vi "Teleop.vi"(10 "Match Info":T1={"Autonomous Elapsed Seconds"=0.0, "TeleOp Elapsed Seconds"=0.0, "Disabled Elapsed Seconds"=0.0, "Visited Autonomous"=FALSE, "Visited TeleOp"=FALSE, "Visited Disabled"=FALSE, "Autonomous Settings"={"Autonomous Style"=enum."Independent", "VI Refnum"=refnum}}, 11 "Call Context":T2) -> ()   [LabVIEW 2011]
doc: "This VI is called for each TeleOp packet received from the DS where the robot is not disabled. It is often used to read from the joysticks and update I/O or to update setpoints for timed control loops. It should complete and return within 20 milliseconds or it may miss DS packets."
uses:
  <vilib>/Rock Robotics/WPI/DriverStation/WPI_DriverStationDerivedRobotMode.ctl
  <vilib>/Rock Robotics/WPI/DriverStation/WPI_DriverStationMatch Info.ctl
  <vilib>/Rock Robotics/WPI/Relay/WPI_RelayValue.ctl
  Robot Global Data.vi
  System Set Points and States.vi
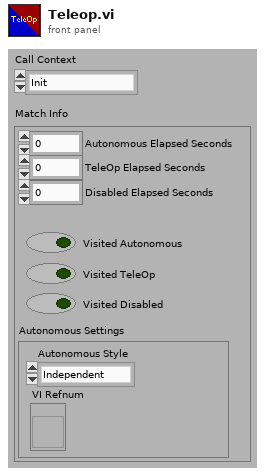
[diagram p1: front panel]
types:
  T1 = typedef "WPI_DriverStationMatch Info.ctl" = cluster{"Autonomous Elapsed Seconds":dbl, "TeleOp Elapsed Seconds":dbl, "Disabled Elapsed Seconds":dbl, "Visited Autonomous":bool, "Visited TeleOp":bool, "Visited Disabled":bool, "Autonomous Settings":cluster{"Autonomous Style":enum16{"Iterative", "Independent"}, "VI Refnum":refnum<vi>}}
  T2 = typedef "WPI_DriverStationDerivedRobotMode.ctl" = enum16{"Init", "Execute", "Stop"}
  T3 = typedef "WPI_JoystickDevRef.ctl" = cluster{"Device":T4}
  T4 = typedef "WPI_JoystickDeviceEnum.ctl" = enum16{"USB 1", "USB 2", "USB 3", "USB 4", "Kinect 1", "Kinect 2"}
  T5 = typedef "WPI_JoystickButtonState.ctl" = cluster{"Button 1":bool, "Button 2":bool, "Button 3":bool, "Button 4":bool, "Button 5":bool, "Button 6":bool, "Button 7":bool, "Button 8":bool, "Button 9":bool, "Button 10":bool, "Button 11":bool, "Button 12":bool}
  T6 = cluster{"axis 1 (x)":dbl, "axis 2 (y)":dbl, "axis 3 (throttle)":dbl, "axis 4":dbl, "axis 5":dbl, "axis 6":dbl}
  T7 = typedef "WPI_RelayValue.ctl" = enum16{"Off", "On", "Forward", "Reverse"}
  T8 = typedef "WPI_DigitalInputDevRef.ctl" = cluster{"DevStatus":errorcluster, "DIO Channel":T9, "Digital Module":T10}
  T9 = typedef "FPGA_DIOChannel.ctl" = enum8{"DIO 1", "DIO 2", "DIO 3", "DIO 4", "DIO 5", "DIO 6", "DIO 7", "DIO 8", "DIO 9", "DIO 10", "DIO 11", "DIO 12", "DIO 13", "DIO 14", "Invalid"}
  T10 = typedef "FPGA_TypedefDigitalModule.ctl" = enum16{"Digital Module 1", "Digital Module 2"}
  T11 = typedef "WPI_RobotDriveDevRef.ctl" = cluster{"DevStatus":errorcluster, "Motors[]":T12[], "Square Inputs":bool, "Max Output":dbl, "Isochronous":bool}
  T12 = typedef "WPI_MotorControlDeviceRef.ctl" = cluster{"DeviceStatus":errorcluster, "Type":enum16{"PWM", "CAN"}, "PWM":cluster{"Digital Module":T10, "PWM Channel":T13, "DeadBand":T14}, "CAN":cluster{"Device Number":u8, "Control Mode":T15, "Semaphore":T16, "Max Vout":dbl}, "Invert":bool, "TransformRef":T17, "InvTransformRef":T17}
  T13 = typedef "FPGA_DIOPWMChannel.ctl" = enum8{"PWM 1", "PWM 2", "PWM 3", "PWM 4", "PWM 5", "PWM 6", "PWM 7", "PWM 8", "PWM 9", "PWM 10", "Invalid"}
  T14 = typedef "WPI_PWMDeadband.ctl" = cluster{"Name":string, "maxPositivePwm":i32, "minPositivePwm":i32, "centerPwm":i32, "maxNegativePwm":i32, "minNegativePwm":i32, "angularRange":u16}
  T15 = typedef "WPI_CANJaguar_ControlMode.ctl" = enum8{"Percent VBus", "Current", "Speed", "Position", "Voltage"}
  T16 = typedef "Semaphore RefNum" = refnum<k1>
  T17 = typedef "WPI_PWMTransform_ConPane.ctl" = refnum<vi>
  T18 = typedef "WPI_AnalogChannelDevRef.ctl" = cluster{"DevStatus":errorcluster, "Analog Module":T19, "Analog Channel":T20}
  T19 = typedef "FPGA_TypedefAnalogModule.ctl" = enum16{"Analog Module 1", "Analog Module 2"}
  T20 = typedef "FPGA_AIChannel.ctl" = enum8{"AI 1", "AI 2", "AI 3", "AI 4", "AI 5", "AI 6", "AI 7", "AI 8", "Invalid"}
  T21 = typedef "WPI_RelayDevRef.ctl" = cluster{"DevStatus":errorcluster, "Relay Channel":T22, "Digital Module":T10, "Relay Direction":T23}
  T22 = typedef "FPGA_DIORelayChannel.ctl" = enum8{"Relay 1", "Relay 2", "Relay 3", "Relay 4", "Relay 5", "Relay 6", "Relay 7", "Relay 8", "Invalid"}
  T23 = typedef "WPI_RelayDirection.ctl" = enum16{"Both directions", "Forward only", "Reverse only"}
  T24 = cluster{"Position":cluster{"X":dbl, "Y":dbl}, "Distance (ft)":dbl}[]
  T25 = cluster{"Target Info[0]":cluster{"Position":cluster{"X":dbl, "Y":dbl}, "Distance (ft)":dbl}, "Target Info[1]":cluster{"Position":cluster{"X":dbl, "Y":dbl}, "Distance (ft)":dbl}, "Target Info[2]":cluster{"Position":cluster{"X":dbl, "Y":dbl}, "Distance (ft)":dbl}, "Target Info[3]":cluster{"Position":cluster{"X":dbl, "Y":dbl}, "Distance (ft)":dbl}, "Target Info[4]":cluster{"Position":cluster{"X":dbl, "Y":dbl}, "Distance (ft)":dbl}, "Target Info[5]":cluster{"Position":cluster{"X":dbl, "Y":dbl}, "Distance (ft)":dbl}, "Target Info[6]":cluster{"Position":cluster{"X":dbl, "Y":dbl}, "Distance (ft)":dbl}, "Target Info[7]":cluster{"Position":cluster{"X":dbl, "Y":dbl}, "Distance (ft)":dbl}, "Target Info[8]":cluster{"Position":cluster{"X":dbl, "Y":dbl}, "Distance (ft)":dbl}}
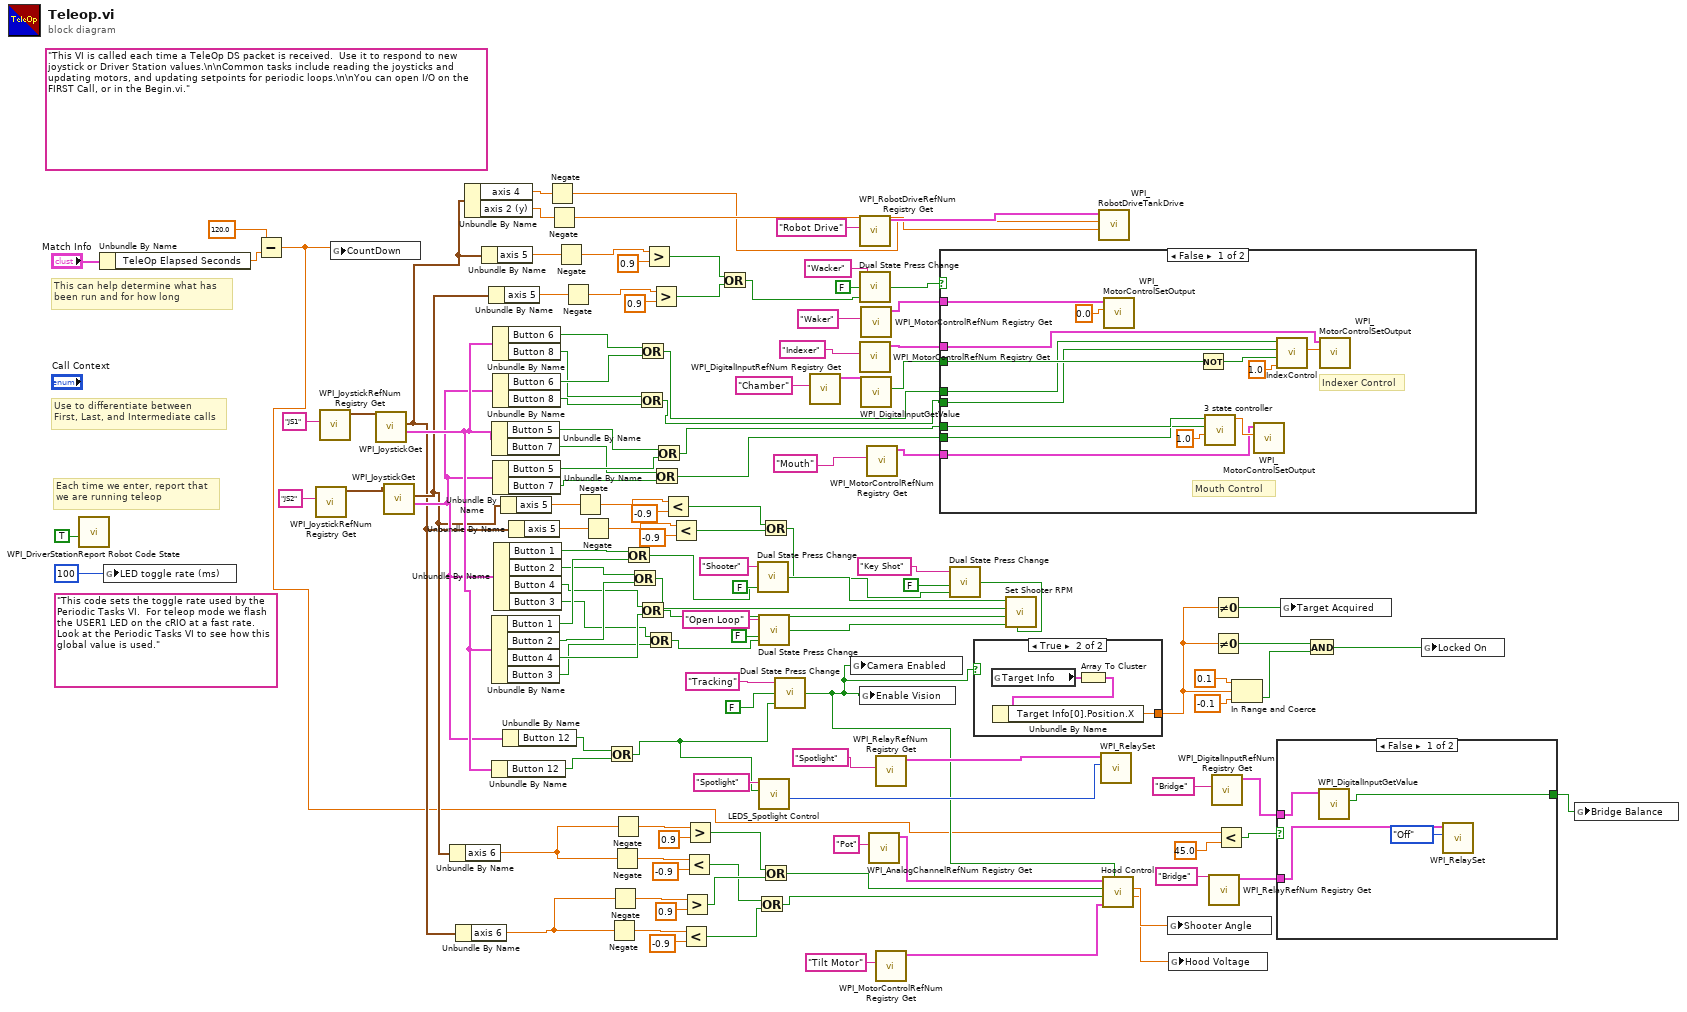
[diagram p0: block diagram]
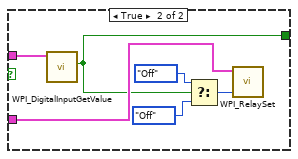
[diagram p2: hidden frame]
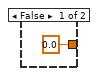
[diagram p3: hidden frame]
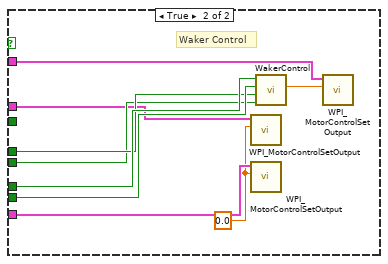
[diagram p4: hidden frame]
diagram:
  (unwired) "This code sets the toggle rate used by the Periodic Tasks VI.  For teleop mode we flash the USER1 LED on the cRIO at a fast rate.  Look at the Periodic Tasks VI to see how this global value is used."
  (unwired) "This VI is called each time a TeleOp DS packet is received.  Use it to respond to new joystick or Driver Station values.\n\nCommon tasks include reading the joysticks and updating motors, and updating setpoints for periodic loops.\n\nYou can open I/O on the FIRST Call, or in the Begin.vi."
  # "Each time we enter, report that\nwe are running teleop"
  # "Use to differentiate between\nFirst, Last, and Intermediate calls"
  # "This can help determine what has\nbeen run and for how long"
  n1 = call <vilib>:"WPI_DriverStationReport Robot Code State.vi"("TeleOp"=TRUE ("Autonomous")) -> ()  [unwired: 10 in, 1 out]
  n2 = Unbundle By Name("Match Info") -> ("TeleOp Elapsed Seconds"=w83:dbl)
  n3 = global write "Robot Global Data.vi" "LED toggle rate (ms)"(u32 100 ("LED ms toggle rate")) -> ()
  n4 = Subtract(x=120.0, y=w83) -> (x-y=w5:dbl)
  n5 = call <vilib>:"WPI_JoystickRefNum Registry Get.vi"("refnum name"="JS2") -> ("JoystickDevRef"=w68:T3)  [unwired: 9 in, 1 out]
  n6 = call <vilib>:"WPI_JoystickRefNum Registry Get.vi"("refnum name"="JS1") -> ("JoystickDevRef"=w125:T3)  [unwired: 9 in, 1 out]
  n7 = global write "System Set Points and States.vi" "CountDown"(w5) -> ()
  n8 = call <vilib>:"WPI_JoystickGet.vi"("JoystickDevRef"=w125) -> ("Buttons"=w97:T5, "Axes"=w13:T6)  [unwired: 4 in, 1 out]
  n9 = call <vilib>:"WPI_JoystickGet.vi"("JoystickDevRef"=w68) -> ("Buttons"=w48:T5, "Axes"=w14:T6)  [unwired: 4 in, 1 out]
  n10 = Unbundle By Name(w14) -> ("axis 6"=w29:dbl)
  n11 = Unbundle By Name(w13) -> ("axis 6"=w75:dbl)
  n12 = Unbundle By Name(w13) -> ("axis 4"=w120:dbl, "axis 2 (y)"=w119:dbl)
  n13 = Unbundle By Name(w13) -> ("axis 5"=w118:dbl)
  n14 = Unbundle By Name(w14) -> ("axis 5"=w42:dbl)
  n15 = Unbundle By Name(w97) -> ("Button 5"=w49:bool, "Button 7"=w45:bool)
  n16 = Unbundle By Name(w97) -> ("Button 1"=w66:bool, "Button 2"=w63:bool, "Button 4"=w61:bool, "Button 3"=w58:bool)
  n17 = Unbundle By Name(w97) -> ("Button 12"=w35:bool)
  n18 = Unbundle By Name(w97) -> ("Button 6"=w54:bool, "Button 8"=w52:bool)
  n19 = Unbundle By Name(w48) -> ("Button 6"=w55:bool, "Button 8"=w51:bool)
  n20 = Unbundle By Name(w48) -> ("Button 5"=w47:bool, "Button 7"=w44:bool)
  n21 = Unbundle By Name(w48) -> ("Button 1"=w67:bool, "Button 2"=w64:bool, "Button 4"=w60:bool, "Button 3"=w57:bool)
  n22 = Unbundle By Name(w14) -> ("axis 5"=w20:dbl)
  n23 = Unbundle By Name(w48) -> ("Button 12"=w36:bool)
  n24 = Unbundle By Name(w13) -> ("axis 5"=w17:dbl)
  n25 = Negate(x=w120) -> (-x=w121:dbl)
  n26 = Negate(x=w119) -> (-x=w122:dbl)
  n27 = Negate(x=w118) -> (-x=w116:dbl)
  n28 = Negate(x=w42) -> (-x=w40:dbl)
  n29 = Negate(x=w20) -> (-x=w18:dbl)
  n30 = Negate(x=w17) -> (-x=w15:dbl)
  n31 = Or(x=w36, y=w35) -> (x .or. y?=w34:bool)
  n32 = Negate(x=w75) -> (-x=w80:dbl)
  n33 = Negate(x=w75) -> (-x=w76:dbl)
  n34 = Negate(x=w29) -> (-x=w32:dbl)
  n35 = Negate(x=w29) -> (-x=w30:dbl)
  n36 = Or(x=w67, y=w66) -> (x .or. y?=w65:bool)
  n37 = Or(x=w64, y=w63) -> (x .or. y?=w62:bool)
  n38 = Or(x=w52, y=w51) -> (x .or. y?=w50:bool)
  n39 = Or(x=w54, y=w55) -> (x .or. y?=w53:bool)
  n40 = Or(x=w60, y=w61) -> (x .or. y?=w59:bool)
  n41 = Greater?(x=w116, y=0.9) -> (0:w38:bool)
  n42 = Or(x=w57, y=w58) -> (x .or. y?=w56:bool)
  n43 = Greater?(x=w40, y=0.9) -> (0:w39:bool)
  n44 = Or(x=w45, y=w44) -> (x .or. y?=w43:bool)
  n45 = Or(x=w49, y=w47) -> (x .or. y?=w46:bool)
  n46 = Less?(x=w18, y=-0.9) -> (x < y?=w12:bool)
  n47 = Less?(x=w15, y=-0.9) -> (x < y?=w11:bool)
  n48 = Less?(x=w80, y=-0.9) -> (x < y?=w25:bool)
  n49 = Greater?(x=w76, y=0.9) -> (0:w27:bool)
  n50 = Less?(x=w32, y=-0.9) -> (x < y?=w26:bool)
  n51 = Greater?(x=w30, y=0.9) -> (0:w28:bool)
  n52 = Or(x=w38, y=w39) -> (x .or. y?=w37:bool)
  n53 = Or(x=w26, y=w25) -> (x .or. y?=w23:bool)
  n54 = call "Dual State Press Change.vi"("Enable/Disable"=w65, "Initial"=FALSE, "Value Name"="Shooter") -> ("Enabled"=w98:bool)
  n55 = call "Dual State Press Change.vi"("Enable/Disable"=w56, "Initial"=FALSE, "Value Name"="Open Loop") -> ("Enabled"=w99:bool)
  n56 = call "LEDS_Spotlight Control.vi"("Name"="Spotlight", "Button"=w34) -> ("Relay State"=w92:T7)  [unwired: 8 in]
  n57 = Or(x=w12, y=w11) -> (x .or. y?=w10:bool)
  n58 = Or(x=w28, y=w27) -> (x .or. y?=w24:bool)
  n59 = call "Dual State Press Change.vi"("Enable/Disable"=w34, "Initial"=FALSE, "Value Name"="Tracking") -> ("Enabled"=w72:bool)
  n60 = call <vilib>:"WPI_DigitalInputRefNum Registry Get.vi"("refnum name"="Chamber") -> ("DigitalInputDevRef"=w106:T8)  [unwired: 9 in, 1 out]
  n61 = global write "System Set Points and States.vi" "Camera Enabled"(w72) -> ()
  n62 = call <vilib>:"WPI_RobotDriveRefNum Registry Get.vi"("refnum name"="Robot Drive") -> ("RobotDriveDevRef"=w123:T11)  [unwired: 9 in, 1 out]
  n63 = call "Dual State Press Change.vi"("Enable/Disable"=w37, "Initial"=FALSE, "Value Name"="Wacker") -> ("Enabled"=w112:bool)
  n64 = call <vilib>:"WPI_MotorControlRefNum Registry Get.vi"("refnum name"="Indexer") -> ("MotorControlDevRef"=w107:T12)  [unwired: 9 in, 1 out]
  n65 = global write "Robot Global Data.vi" "Enable Vision"(w72) -> ()
  n66 = call <vilib>:"WPI_MotorControlRefNum Registry Get.vi"("refnum name"="Waker") -> ("MotorControlDevRef"=w109:T12)  [unwired: 9 in, 1 out]
  n67 = call <vilib>:"WPI_DigitalInputGetValue.vi"("DigitalInputDevRef"=w106) -> ("Value"=w104:bool)  [unwired: 8 in, 2 out]
  n68 = call <vilib>:"WPI_MotorControlRefNum Registry Get.vi"("refnum name"="Mouth") -> ("MotorControlDevRef"=w113:T12)  [unwired: 9 in, 1 out]
  n69 = call <vilib>:"WPI_AnalogChannelRefNum Registry Get.vi"("refnum name"="Pot") -> ("AIDeviceRef"=w73:T18)  [unwired: 9 in, 1 out]
  n70 = call <vilib>:"WPI_RelayRefNum Registry Get.vi"("refnum name"="Spotlight") -> ("RelayDevRef"=w94:T21)  [unwired: 9 in, 1 out]
  n71 = call <vilib>:"WPI_MotorControlRefNum Registry Get.vi"("refnum name"="Tilt Motor") -> ("MotorControlDevRef"=w74:T12)  [unwired: 9 in, 1 out]
  n72 = case shown="False" w112 {
    tunnel: w46 -> [w139 w151]
    tunnel: w43 -> [w138 w150]
    tunnel: w53 -> [w131 w149]
    tunnel: w50 -> [w130 w148]
    tunnel: w113 -> [w137 w145]
    tunnel: w107 -> [w136 w146]
    tunnel: w109 -> [w135 w147]
    tunnel: w104 -> [w133 _]
    frame False {
      # "Indexer Control"
      # "Mouth Control"
      n73 = call <vilib>:"WPI_MotorControlSetOutput.vi"("Output"=0.0, "MotorControlDevRef"=w135) -> ()  [unwired: 8 in, 2 out]
      n74 = Not(x=w133) -> (.not. x?=w132:bool)
      n75 = call "3 state controller.vi"("Power"=1.0, "Backward"=w138, "Forward"=w139) -> ("Numeric"=w143:dbl)  [unwired: 8 in]
      n76 = call <vilib>:"WPI_MotorControlSetOutput.vi"("Output"=w143, "MotorControlDevRef"=w137) -> ()  [unwired: 8 in, 2 out]
      n77 = call "IndexControl.vi"("Power"=1.0, "Chamber"=w132, "Back"=w130, "Forward"=w131) -> ("Numeric"=w141:dbl)  [unwired: 7 in]
      n78 = call <vilib>:"WPI_MotorControlSetOutput.vi"("Output"=w141, "MotorControlDevRef"=w136) -> ()  [unwired: 8 in, 2 out]
    }
    frame True {
      w144 = 0.0 ("Output")
      # "Waker Control"
      n79 = call <vilib>:"WPI_MotorControlSetOutput.vi"("Output"=w144, "MotorControlDevRef"=w146) -> ()  [unwired: 8 in, 2 out]
      n80 = call <vilib>:"WPI_MotorControlSetOutput.vi"("Output"=w144, "MotorControlDevRef"=w145) -> ()  [unwired: 8 in, 2 out]
      n81 = call "WakerControl.vi"("Button 4"=w148, "Button 2"=w149, "Button 3"=w150, "Button 1"=w151) -> ("Speed Out"=w152:dbl)  [unwired: 5 in]
      n82 = call <vilib>:"WPI_MotorControlSetOutput.vi"("Output"=w152, "MotorControlDevRef"=w147) -> ()  [unwired: 8 in, 2 out]
    }
  }
  n83 = call "Dual State Press Change.vi"("Enable/Disable"=w10, "Initial"=FALSE, "Value Name"="Key Shot") -> ("Enabled"=w9:bool)
  n84 = case shown="True" w72 {
    tunnel: [0.0 ("Distance (ft)") w154] -> w84
    frame False {
    }
    frame True {
      n85 = global read "Robot Global Data.vi" "Target Info"() -> (w156:T24)
      n86 = Array To Cluster(array=w156) -> (cluster=w155:T25)
      n87 = Unbundle By Name(w155) -> ("Target Info[0].Position.X"=w154:dbl)
    }
  }
  n88 = call "Set Shooter RPM.vi"("Key Shot"=w9, "Open Loop"=w99, "Increment"=w59, "Decrement"=w62, "Shooter Enabled"=w98) -> ()  [unwired: 7 in]
  n89 = call <vilib>:"WPI_RobotDriveTankDrive.vi"("Right axis value"=w122, "Left axis value"=w121, "RobotDriveDevRef"=w123) -> ()  [unwired: 7 in, 2 out]
  n90 = call <vilib>:"WPI_RelaySet.vi"("RelayValue"=w92, "RelayDevRef"=w94) -> ()  [unwired: 8 in, 2 out]
  n91 = call "Hood Control.vi"("Vision"=w72, "MotorControlDevRef"=w74, "Down"=w23, "Up"=w24, "AIDeviceRef"=w73) -> ("Voltage"=w70:dbl, "Shoter Angle"=w71:dbl)  [unwired: 5 in]
  n92 = global write "System Set Points and States.vi" "Shooter Angle"(w71) -> ()
  n93 = global write "System Set Points and States.vi" "Hood Voltage"(w70) -> ()
  n94 = call <vilib>:"WPI_RelayRefNum Registry Get.vi"("refnum name"="Bridge") -> ("RelayDevRef"=w3:T21)  [unwired: 9 in, 1 out]
  n95 = call <vilib>:"WPI_DigitalInputRefNum Registry Get.vi"("refnum name"="Bridge") -> ("DigitalInputDevRef"=w8:T8)  [unwired: 9 in, 1 out]
  n96 = Not Equal To 0?(x=w84) -> (x != 0?=w88:bool)
  n97 = Not Equal To 0?(x=w84) -> (x != 0?=w87:bool)
  n98 = Less?(x=w5, y=45.0) -> (x < y?=w6:bool)
  n99 = In Range and Coerce(upper limit=0.1, x=w84, lower limit=-0.1) -> (In Range?=w86:bool)  [unwired: 1 out]
  n100 = case shown="False" w6 {
    tunnel: w8 -> [w158 w166]
    tunnel: w3 -> [w160 w162]
    tunnel: [w157 w161] -> w1
    frame False {
      n101 = call <vilib>:"WPI_DigitalInputGetValue.vi"("DigitalInputDevRef"=w158) -> ("Value"=w157:bool)  [unwired: 8 in, 2 out]
      n102 = call <vilib>:"WPI_RelaySet.vi"("RelayValue"=WPI_RelayValue."Off", "RelayDevRef"=w160) -> ()  [unwired: 8 in, 2 out]
    }
    frame True {
      n103 = call <vilib>:"WPI_DigitalInputGetValue.vi"("DigitalInputDevRef"=w166) -> ("Value"=w161:bool)  [unwired: 8 in, 2 out]
      n104 = Select(t=WPI_RelayValue."Off" ("Relay State"), s=w161, f=WPI_RelayValue."Off" ("Relay State")) -> (s? t:f=w165:T7)
      n105 = call <vilib>:"WPI_RelaySet.vi"("RelayValue"=w165, "RelayDevRef"=w162) -> ()  [unwired: 8 in, 2 out]
    }
  }
  n106 = global write "System Set Points and States.vi" "Target Acquired"(w88) -> ()
  n107 = And(x=w87, y=w86) -> (x .and. y?=w85:bool)
  n108 = global write "System Set Points and States.vi" "Locked On"(w85) -> ()
  n109 = global write "System Set Points and States.vi" "Bridge Balance"(w1) -> ()
